vi "Platform by Name.vi"(8 "error in (no error)":errorcluster, 10 "Platform":string, 11 "TargetPluginManager in":refnum<class "PlatformPluginManager.lvclass">) -> (0 "error out":errorcluster, 2 "Target":refnum<class "DeployPlatform.lvclass">, 3 "TargetPluginManager out":refnum<class "PlatformPluginManager.lvclass">)   [LabVIEW 2020, in "PicoG-Core.lvlib" / "PlatformPluginManager.lvclass"]
uses:
  PlatformPluginManager.lvclass
  DeployPlatform/DeployPlatform.lvclass
  PlatformPluginManager.lvclass/PlatformPluginManager.ctl
  <vilib>/Utility/error.llb/Error Cluster From Error Code.vi
  <vilib>/ErrorRing/Error Ring.xnode
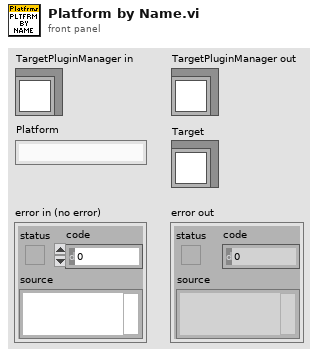
[diagram p1: front panel]
types:
  T1 = typedef "PicoG-Core.lvlib/PlatformPluginManager.lvclass/Ref Data.ctl" = cluster{"Platforms":refnum<class "DeployPlatform.lvclass">[], "Last Platform":refnum<class "DeployPlatform.lvclass">, "Last Resource":refnum<class "DeployResource.lvclass">}
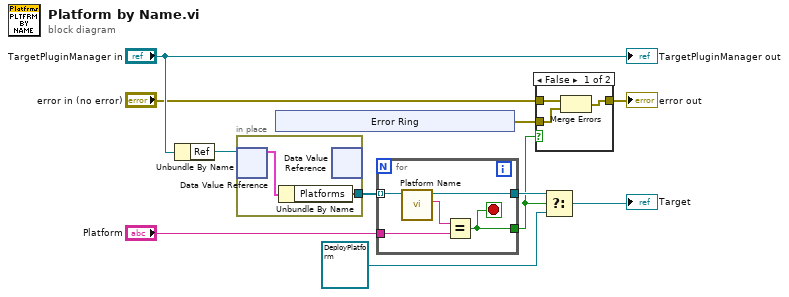
[diagram p0: block diagram]
diagram:
  n1 = Unbundle By Name("TargetPluginManager in") -> ("Ref"=w11:refnum<data-value>)
  n2 = in-place {
    in-place-border: [w12] -> w9
    n3 = in-place-dvr #1(w11) -> (w13:T1)  [unwired: 1 out]
    n4 = Unbundle By Name(w13) -> ("Platforms"=w12:refnum<class "DeployPlatform.lvclass">[])
    n5 = in-place-dvr #1() -> ()  [unwired: 1 in, 2 out]
  }
  n6 = xnode "Error Ring"() -> ("error out"=w3:errorcluster)
  n7 = for {
    tunnel: w9 -> [w18] mode=indexing
    tunnel: "Platform" -> [w17]
    tunnel: [w15] -> w7
    tunnel: [w14] -> w4
    stop <- w14 stop-if-true
    n8 = call-dynamic "Platform Name.vi"("DeployTarget in"=w18) -> ("Platform Name"=w16:string, "DeployTarget out"=w15:refnum<class "DeployPlatform.lvclass">)  [unwired: 8 in, 1 out]
    n9 = Equal?(x=w16, y=w17) -> (x = y?=w14:bool)
  }
  n10 = case shown="False" w4 {
    tunnel: w3 -> [w20 _]
    tunnel: "error in (no error)" -> [w21 w22]
    tunnel: [w19 w22] -> w1
    frame False {
      n11 = Merge Errors(w21, w20) -> (w19:errorcluster)
    }
    frame True {
    }
  }
  "error out" <- w1
  n12 = Select(t=w7, s=w4, f=refnum<class "DeployPlatform.lvclass"> refnum) -> (s? t:f=→"Target":refnum<class "DeployPlatform.lvclass">)
  "TargetPluginManager out" <- "TargetPluginManager in"
